vi "Profile Step 2 Parameters.vi"(7 "Profile Step":string[](array[string])) -> (4 "Parameter 1":i32, 6 "Setpoint 1":dbl format="%#_13g", 8 "Parameter 2":i32, 10 "Setpoint 2":dbl format="%#_13g", 15 "Setpoint 3":dbl format="%#_13g")   [LabVIEW 2013]
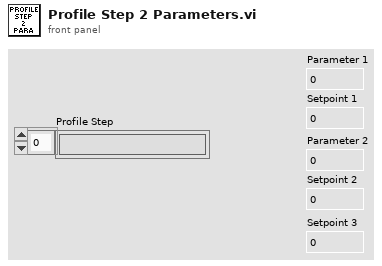
[diagram p1: front panel]
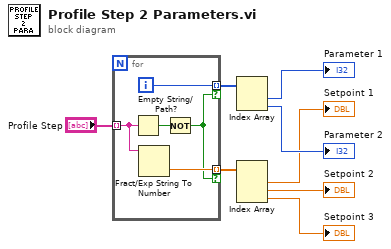
[diagram p0: block diagram]
diagram:
  n1 = for {
    tunnel: "Profile Step" -> [w11] mode=indexing
    tunnel: [w12] -> w7 mode=indexing if=w9
    tunnel: [w10] -> w6 mode=indexing if=w9
    i -> [w12]
    n2 = Empty String/Path?(string/path=w11) -> (empty?=w13:bool)
    n3 = Fract/Exp String To Number(string=w11) -> (number=w10:dbl)  [unwired: 3 in, 1 out]
    n4 = Not(x=w13) -> (.not. x?=w9:bool)
  }
  n5 = Index Array(array=w7) -> (element #1=→"Parameter 1":i32, element #2=→"Parameter 2":i32)  [unwired: 2 in]
  n6 = Index Array(array=w6) -> (element #1=→"Setpoint 1":dbl, element #2=→"Setpoint 2":dbl, element #3=→"Setpoint 3":dbl)  [unwired: 3 in]
